vi "YPR_SubVI_string.vi"(11 "read buffer":string) -> (1 "Roll":sgl format="%#_10g", 2 "Pitch":sgl format="%#_10g", 3 "Yaw":sgl format="%#_10g")   [LabVIEW 2016]
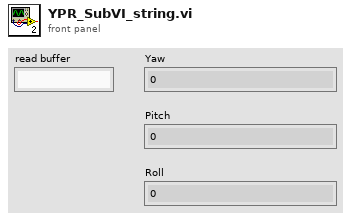
[diagram p1: front panel]
types:
  T1 = enum16{"big-endian, network order", "native, host order", "little-endian"}
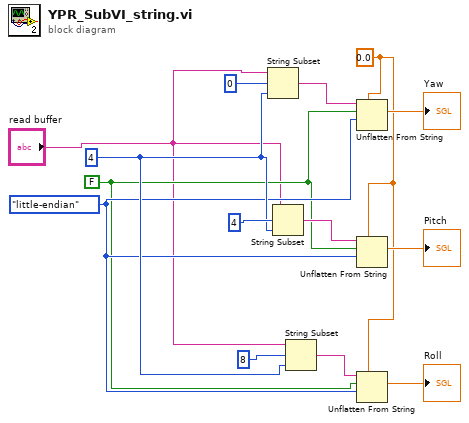
[diagram p0: block diagram]
diagram:
  w2 = sgl 0.0
  w3 = FALSE ("data includes array or string size? (T)")
  w4 = T1."little-endian" ("byte order (0:big-endian, network order)")
  w5 = 4
  n1 = String Subset(string="read buffer", offset (0)=0, length (rest)=w5) -> (substring=w8:string)
  n2 = String Subset(string="read buffer", offset (0)=4, length (rest)=w5) -> (substring=w11:string)
  n3 = String Subset(string="read buffer", offset (0)=8, length (rest)=w5) -> (substring=w14:string)
  n4 = Unflatten From String(type=w2, binary string=w8, data includes array or string size? (T)=w3, byte order (0:big-endian, network order)=w4) -> (value=→"Yaw":sgl)  [unwired: 1 in, 2 out]
  n5 = Unflatten From String(type=w2, binary string=w11, data includes array or string size? (T)=w3, byte order (0:big-endian, network order)=w4) -> (value=→"Pitch":sgl)  [unwired: 1 in, 2 out]
  n6 = Unflatten From String(type=w2, binary string=w14, data includes array or string size? (T)=w3, byte order (0:big-endian, network order)=w4) -> (value=→"Roll":sgl)  [unwired: 1 in, 2 out]
